vi "FTW-Container-Element-Get.vi"(0 "FTW-Container In":refnum<class "FTW-Container.lvclass">, 5 "Element Name":string, 7 "Default Value":variant, 9 "Delete?":bool, 11 "error in":errorcluster) -> (4 "FTW-Container Out":refnum<class "FTW-Container.lvclass">, 6 "Element Out":refnum<class "FTW-Container.lvclass">, 8 "Found":bool, 15 "error out":errorcluster)   [LabVIEW 2015, in "FTW-Container.lvclass"]
uses:
  FTW-Container.lvclass
  FTW-Container.lvclass/FTW-Container.ctl
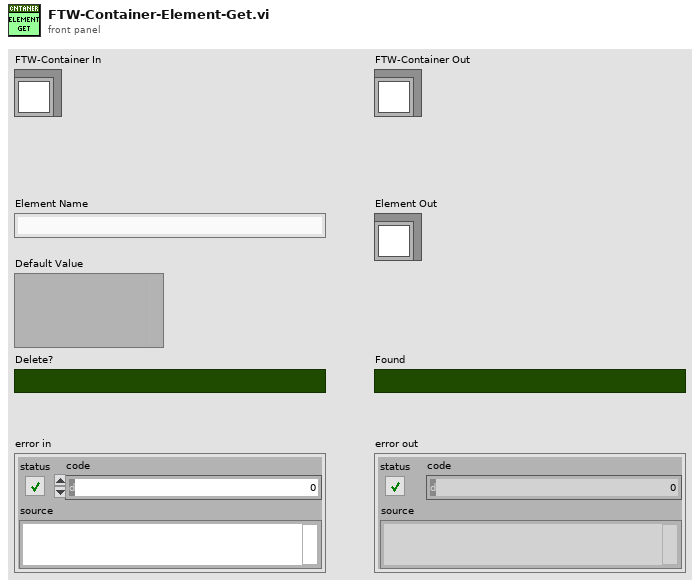
[diagram p1: front panel]
types:
  T1 = typedef "FTW-Container.lvclass/FTW-Container-Object.ctl" = cluster{"Names":string[], "Values":variant[]}
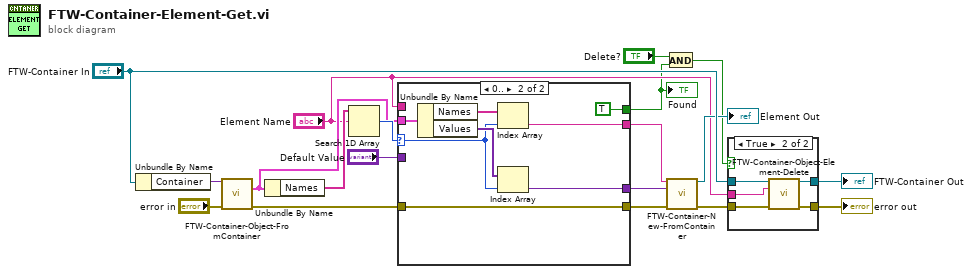
[diagram p0: block diagram]
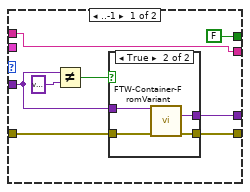
[diagram p2: hidden frame]
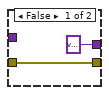
[diagram p3: hidden frame]
diagram:
  n1 = Unbundle By Name("FTW-Container In") -> ("Container"=w15:variant)
  n2 = call "FTW-Container-Object-FromContainer.vi"("FTW-Container In"=w15, "error in"="error in") -> (6:w12:T1, "error out"=w6:errorcluster)  [unwired: 12 in]
  n3 = Unbundle By Name(w12) -> ("Names"=w14:string[])
  n4 = Search 1D Array(1D array=w14, element="Element Name") -> (index of element=w13:i32)  [unwired: 1 in]
  n5 = case shown="0.." w13 {
    selector: w13 -> [_ w34]
    tunnel: [FALSE TRUE] -> w4
    tunnel: w12 -> [_ w40]
    tunnel: [w26 w37] -> w11
    tunnel: [w23 w36] -> w10
    tunnel: "Default Value" -> [w22 _]
    tunnel: "Element Name" -> [w26 _]
    tunnel: w6 -> [w25 w35]
    tunnel: [w24 w35] -> w2
    frame ..-1 {
      n6 = Not Equal?(x=w22, y=variant) -> (x != y?=w20:bool)
      n7 = case shown="True" w20 {
        tunnel: w22 -> [_ w33]
        tunnel: w25 -> [w28 w32]
        tunnel: [w28 w31] -> w24
        tunnel: [variant w30] -> w23
        frame False {
        }
        frame True {
          n8 = call "FTW-Container-FromVariant.vi"("Variant"=w33, "error in"=w32) -> ("Container"=w30:variant, "error out"=w31:errorcluster)  [unwired: 11 in, 1 out]
        }
      }
    }
    frame 0.. {
      n9 = Unbundle By Name(w40) -> ("Names"=w39:string[], "Values"=w38:variant[])
      n10 = Index Array(array=w39, index=w34) -> (element=w37:string)
      n11 = Index Array(array=w38, index=w34) -> (element=w36:variant)
    }
  }
  "Found" <- w4
  n12 = And(x="Delete?", y=w4) -> (x .and. y?=w5:bool)
  n13 = call "FTW-Container-New-FromContainer.vi"("Name"=w11, "Container"=w10, "error in"=w2) -> ("FTW-Container"=→"Element Out":refnum<class "FTW-Container.lvclass">, "error out"=w1:errorcluster)  [unwired: 11 in]
  n14 = case shown="True" w5 {
    tunnel: [w43 w48] -> w3
    tunnel: [w42 w47] -> w19
    tunnel: w1 -> [w43 w46]
    tunnel: "FTW-Container In" -> [w42 w45]
    tunnel: "Element Name" -> [_ w44]
    frame False {
    }
    frame True {
      n15 = call "FTW-Container-Object-Element-Delete.vi"("FTW-Container In"=w45, "Element Name"=w44, "error in"=w46) -> ("FTW-Container Out"=w47:refnum<class "FTW-Container.lvclass">, "error out"=w48:errorcluster)  [unwired: 10 in, 1 out]
    }
  }
  "error out" <- w3
  "FTW-Container Out" <- w19
